vi "Celda solar Tiempo Real.vi"() -> ()   [LabVIEW 2014]
uses:
  <vilib>/imath/engines/lvmath2/RunTimeEngine/ArithmeticOperatorToken/NIMS_ArithmeticOperator_power(S).vi
  <instcachedir>/0/NIMS_ArithmeticOperator_power(S)_CAFE680B12A64A3A8F5E28A20C679B7D.lvgen/NIMS_ArithmeticOperator_power(S)_CAFE680B12A64A3A8F5E28A20C679B7D_014.vi
  <vilib>/imathl/engines/lvmath/Functions/Error Handling/Create Error.vi
  <vilib>/imath/engines/lvmath2/RunTimeEngine/CommandStatement/MC_CommandStatement_break.vi
  <vilib>/imath/engines/lvmath2/RunTimeEngine/RangeToken/NIMS_Range_R2 - Integer.vi
  <instcachedir>/0/NIMS_Range_R2 - Integer_2D1304BAF97744E0A293025746CBADFC.lvgen/NIMS_Range_R2 - Integer_2D1304BAF97744E0A293025746CBADFC_000.vi
  <vilib>/imath/engines/lvmath2/RunTimeEngine/IndexReplace/NIMS V(S)=S.vi
  <instcachedir>/0/NIMS V(S)=S_2D52C4EC15D8415E870AEE69FB516CCA.lvgen/NIMS V(S)=S_2D52C4EC15D8415E870AEE69FB516CCA_001.vi
  <instcachedir>/0/NIMS V(S)=S_2D52C4EC15D8415E870AEE69FB516CCA.lvgen/NIMS V(S)=S_2D52C4EC15D8415E870AEE69FB516CCA_000.vi
  <vilib>/imath/engines/lvmath2/RunTimeEngine/CommandStatement/NIMS_CommandStatement_MaskErr.vi
  <vilib>/imath/engines/lvmath2/RunTimeEngine/NodeEndStatement/NIMS_NodeEndStatement_Output.vi
  <instcachedir>/0/NIMS_NodeEndStatement_Output_53EC0D466D134D7ABD903AC30B43404B.lvgen/NIMS_NodeEndStatement_Output_53EC0D466D134D7ABD903AC30B43404B_000.vi
  <instcachedir>/0/NIMS_NodeEndStatement_Output_53EC0D466D134D7ABD903AC30B43404B.lvgen/NIMS_NodeEndStatement_Output_53EC0D466D134D7ABD903AC30B43404B_005.vi
  <vilib>/imath/engines/lvmath2/RunTimeEngine/ErrorHandling/NIMS_Finalize Error.vi
panel:
  out "Voltaje maximo":dbl
  out "Potencia Maxima":sgl
  out "x*y":cdb[](array[numeric])
  in  "Tab Control":enum32{"Page 2"}(tab)
  in  "Retraso (ms)":i32(slide) scale=0.0..500.0
  in  "Resistencia de carga":dbl
  out "Curva de Potencia":cluster{dbl[], sgl[]}(graph)
  in  "Configuracion":enum32{"Predeterminado", "Avanzado"}(tab)
  out "Factor de calidad":dbl=1.2
  out "T1":dbl=1.2
  out "Voc T1":dbl=1.2
  out "Isc T1":dbl=1.2
  out "T2":dbl=1.2
  out "Voc T2":dbl=1.2
  out "Isc T2":dbl=1.2
  in  "Principales Marcas":u16(ring) items=["Solarex MSX60", "Jinko Solar Perc 60-JKM300M-60", "Suntech STP275S-20", "Trina Solar TSM-250PD05", "Canadian Solar CS6X-305P", "JA Solar JAM6 PR mono 60", "Hanwha Q.Peak-G4.1", "Sharp ND-F2Q235", "Yingli YGE Serie YL275P-29b", "SolarWorld SW290", "Kyocera KD265GX-LFB\""]
  out "Vg":dbl=1.2
  out "Celdas en serie":dbl
  in  "Factor de calidad":dbl
  in  "Vg":dbl
  in  "T1":dbl
  in  "Voc T1":dbl
  in  "Isc T1":dbl
  in  "T2":dbl
  in  "Voc T2":dbl
  in  "Isc T2":dbl
  in  "Celdas en series":dbl
  out "Curva Caracteristica I-V":cluster{"Vao":dbl[], "Iao":dbl[]}[](graph)
  out "?":string
  in  "stop":bool
  in  "Paneles en serie":dbl min=1.0
  in  "Paneles en paralelo":dbl min=1.0
  in  "Fecha inicial":timestamp format="%<%Y/%m/%d>T"
  in  "Fecha final":timestamp format="%<%Y/%m/%d>T"
  in  "Latitud":string="10.41"
  in  "Longitud":string="-66.88"
  in  "OK Button":bool
  out "modelo":string
  out "String":string
  out "Numeric":i32
  out "Ia":cdb[](array[numeric])
  # "Curva 1: curva característica del panel solar\n\nCurva 2: recta de carga"
  # "Curva 1: curva de potencia del panel solar"
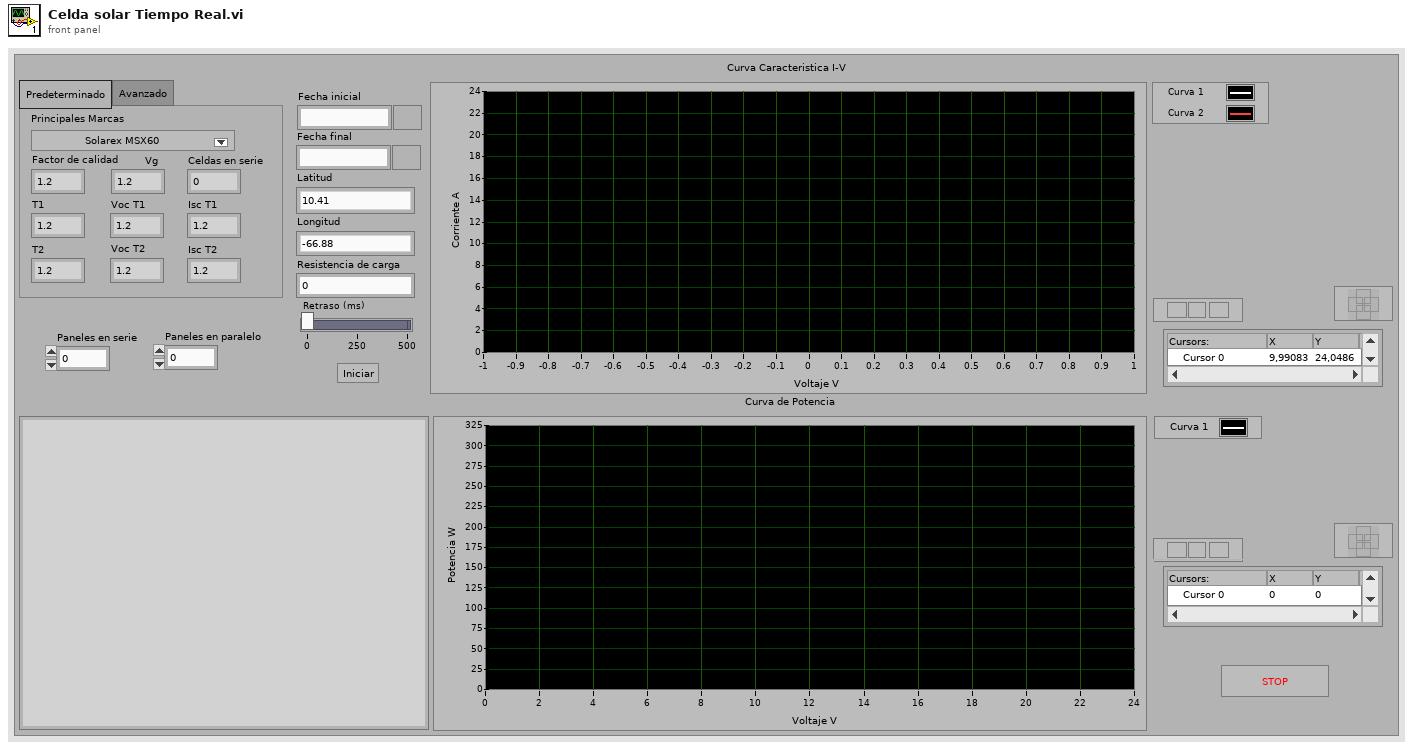
[diagram p1: front panel]
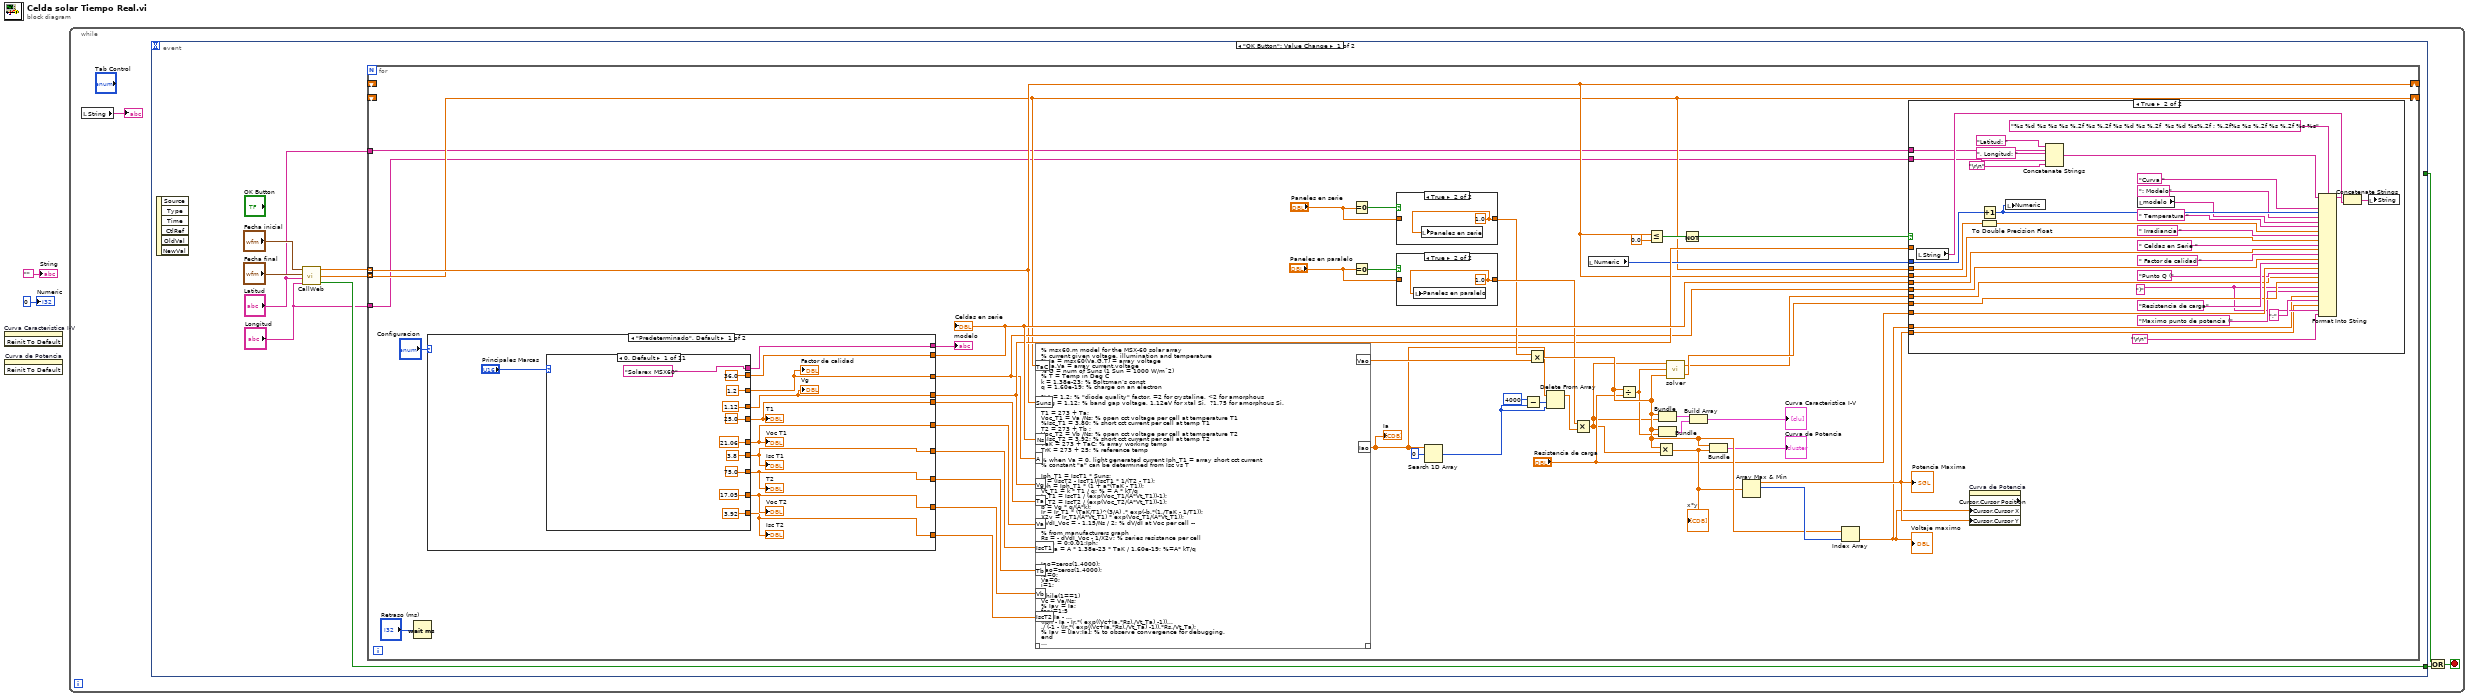
[diagram p0: block diagram]
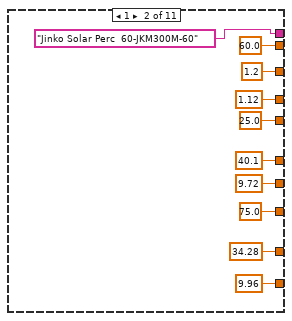
[diagram p4: hidden frame]
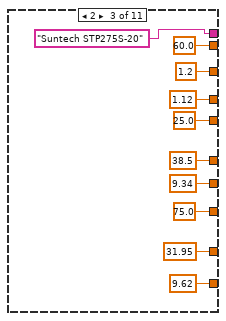
[diagram p5: hidden frame]
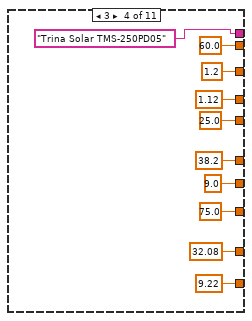
[diagram p6: hidden frame]
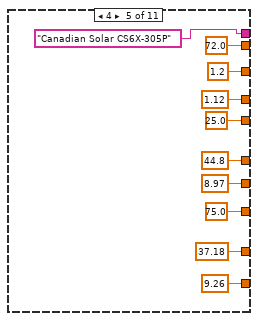
[diagram p7: hidden frame]
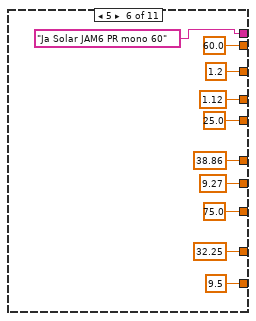
[diagram p8: hidden frame]
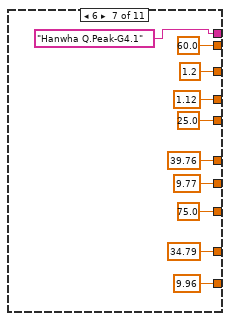
[diagram p9: hidden frame]
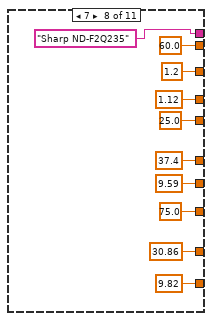
[diagram p10: hidden frame]
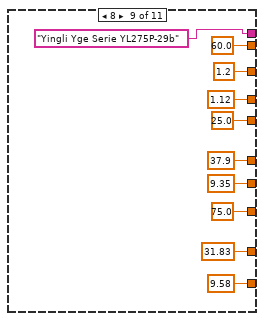
[diagram p11: hidden frame]
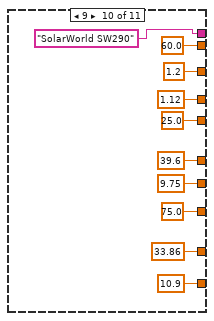
[diagram p12: hidden frame]
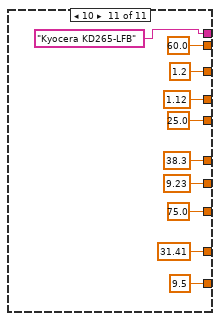
[diagram p13: hidden frame]
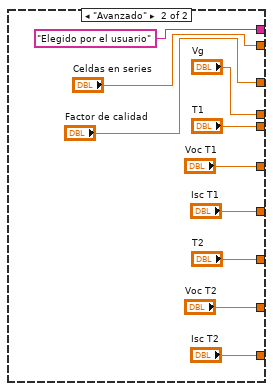
[diagram p14: hidden frame]
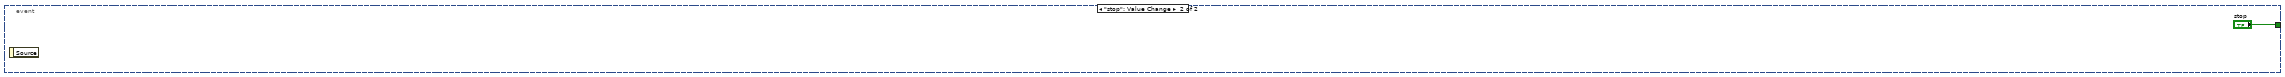
[diagram p16: hidden frame]
diagram:
  n1 = invoke on="Curva Caracteristica I-V" class="XYGraph (strict)" method="Reinit To Default"() -> ()  [unwired: 3 in, 3 out]
  n2 = invoke on="Curva de Potencia" class="XYGraph (strict)" method="Reinit To Default"() -> ()  [unwired: 3 in, 3 out]
  n3 = while {
    stop <- w4 stop-if-true
    n4 = local read "String"() -> (→"?":string)
    n5 = event shown="[0] \"OK Button\": Value Change" {
      selector: _ -> [_ _]
      dyn-events: _ -> [_ _]
      timeout: _ -> [_ _]
      tunnel: [_ "stop"] -> w6
      tunnel: [w9 _] -> w5
      event "OK Button": Value Change {
        n6 = event-data() -> ()  [unwired: 1 in, 6 out]
        n7 = call "CallWeb.vi"("Longitud"="Longitud", "Latitud"="Latitud", "Fecha final"="Fecha final", "Fecha inicial"="Fecha inicial") -> ("error?"=w9:bool, "temperatura"=w10:dbl[], "irradiancia"=w11:dbl[])  [unwired: 1 out]
        n8 = for {
          tunnel: w11 -> [w18] mode=indexing
          shift-right: [w17] -> _
          shift-left: _ -> [_]
          shift-right: [w18] -> _
          shift-left: _ -> [_]
          tunnel: w10 -> [w17] mode=indexing
          tunnel: "Latitud" -> [w15]
          tunnel: "Longitud" -> [w14]
          n9 = Wait (ms)(milliseconds to wait="Retraso (ms)") -> ()  [unwired: 1 out]
          n10 = case shown="\"Predeterminado\", Default" "Configuracion" {
            tunnel: [w74 "Factor de calidad"] -> w26
            tunnel: [w73 "Vg"] -> w27
            tunnel: [w72 "T1"] -> w32
            tunnel: [w71 "Voc T1"] -> w28
            tunnel: [w70 "Isc T1"] -> w33
            tunnel: [w69 "T2"] -> w29
            tunnel: [w68 "Voc T2"] -> w30
            tunnel: [w67 "Isc T2"] -> w31
            tunnel: [w66 "Celdas en series"] -> w60
            tunnel: [w65 "Elegido por el usuario"] -> w35
            frame "Predeterminado", Default {
              n11 = case shown="0, Default" "Principales Marcas" {
                tunnel: [1.2 1.2 1.2 1.2 1.2 1.2 1.2 1.2 1.2 1.2 1.2] -> w74
                tunnel: [1.12 1.12 1.12 1.12 1.12 1.12 1.12 1.12 1.12 1.12 1.12] -> w73
                tunnel: [25.0 25.0 25.0 25.0 25.0 25.0 25.0 25.0 25.0 25.0 25.0] -> w72
                tunnel: [21.06 40.1 38.5 38.2 44.8 38.86 39.76 37.4 37.9 39.6 38.3] -> w71
                tunnel: [3.8 9.72 9.34 9.0 8.97 9.27 9.77 9.59 9.35 9.75 9.23] -> w70
                tunnel: [75.0 75.0 75.0 75.0 75.0 75.0 75.0 75.0 75.0 75.0 75.0] -> w69
                tunnel: [17.05 34.28 31.95 32.08 37.18 32.25 34.79 30.86 31.83 33.86 31.41] -> w68
                tunnel: [3.92 9.96 9.62 9.22 9.26 9.5 9.96 9.82 9.58 10.9 9.5] -> w67
                tunnel: [36.0 60.0 60.0 60.0 72.0 60.0 60.0 60.0 60.0 60.0 60.0] -> w66
                tunnel: ["Solarex MSX60" "Jinko Solar Perc  60-JKM300M-60" "Suntech STP275S-20" "Trina Solar TMS-250PD05" "Canadian Solar CS6X-305P" "Ja Solar JAM6 PR mono 60" "Hanwha Q.Peak-G4.1" "Sharp ND-F2Q235" "Yingli Yge Serie YL275P-29b" "SolarWorld SW290" "Kyocera KD265-LFB"] -> w65
                frame 0, Default {
                }
                frame 1 {
                }
                frame 2 {
                }
                frame 3 {
                }
                frame 4 {
                }
                frame 5 {
                }
                frame 6 {
                }
                frame 7 {
                }
                frame 8 {
                }
                frame 9 {
                }
                frame 10 {
                }
              }
              "Factor de calidad" <- w74
              "Vg" <- w73
              "T1" <- w72
              "Voc T1" <- w71
              "Isc T1" <- w70
              "T2" <- w69
              "Voc T2" <- w68
              "Isc T2" <- w67
            }
            frame "Avanzado" {
            }
          }
          "Celdas en serie" <- w60
          "modelo" <- w35
          n12 = mathscript code="% msx60.m model for the MSX-60 solar array\n% current given voltage, illumination and temperature\n% Ia = msx60(Va,G,T) = array voltage\n% Ia,Va = array current,voltage\n% G = num of Suns (1 Sun = 1000 W/mˆ2)\n% T = Temp in Deg C\nk = 1.38e-23; % Boltzman’s const\nq = 1.60e-19; % charge on an electron\n\n%A = 1.2; % \"diode quality\" factor, =2 for crystaline, <2 for amorphous\n%Vg = 1.12; % band gap voltage, 1.12eV for xtal Si,  ?1.75 for amorphous Si.\n\nT1 = 273 + Ta;\nVoc_T1 = Va /Ns; % open cct voltage per cell at temperature T1\n%Isc_T1 = 3.80; % short cct current per cell at temp T1\nT2 = 273 + Tb ;\nVoc_T2 = Vb /Ns; % open cct voltage per cell at temperature T2\n%Isc_T2 = 3.92; % short cct current per cell at temp T2\nTaK = 273 + TaC; % array working temp\nTrK = 273 + 25; % reference temp\n\n% when Va = 0, light generated current Iph_T1 = array short cct current\n% constant \"a\" can be determined from Isc vs T\n\nIph_T1 = IscT1 * Suns;\na = (IscT2 - IscT1)/IscT1 * 1/(T2 - T1);\nIph = Iph_T1 * (1 + a*(TaK - T1));\nVt_T1 = k * T1 / q; % = A * kT/q\nIr_T1 = IscT1 / (exp(Voc_T1/(A*Vt_T1))-1);\nIr_T2 = IscT2 / (exp(Voc_T2/(A*Vt_T1))-1);\nb = Vg * q/(A*k);\nIr = Ir_T1 * (TaK/T1)^(3/A) .* exp(-b.*(1./TaK - 1/T1));\nX2v = Ir_T1/(A*Vt_T1) * exp(Voc_T1/(A*Vt_T1));\ndVdI_Voc = - 1.15/Ns / 2; % dV/dI at Voc per cell --\n\n% from manufacturers graph\nRs = - dVdI_Voc - 1/X2v; % series resistance per cell\n% Ia = 0:0.01:Iph;\nVt_Ta = A * 1.38e-23 * TaK / 1.60e-19; %=A* kT/q\n\n\nIao=zeros(1,4000);\nVao=zeros(1,4000);\nIa=0;\nVa=0;\ni=1;\n\nwhile(1==1)\nVc = Va/Ns;\n% Iav = Ia;\nfor j=1:5\nIa= Ia - ...\n(Iph - Ia - Ir.*( exp((Vc+Ia.*Rs)./Vt_Ta) -1))...\n./ (-1 - (Ir.*( exp((Vc+Ia.*Rs)./Vt_Ta) -1)).*Rs./Vt_Ta);\n% Iav = [Iav;Ia]; % to observe convergence for debugging.\nend\n\nif(Ia<=0) break\nend\n\nIao(i)=Ia;\nVao(i)=Va;\n\ni=i+1;\nVa=Va+1/100;\n\nend"("TaC"=w17, "Suns"=w18, "Ns"=w60, "Vg"=w27, "A"=w26, "Ta"=w32, "Va"=w28, "IscT1"=w33, "Tb"=w29, "Vb"=w30, "IscT2"=w31) -> ("Iao"=w36:cdb[], "Vao"=w38:dbl[])  [unwired: 1 in, 1 out]
          "Ia" <- w36
          n13 = Equal To 0?(x="Paneles en serie") -> (x = 0?=w39:bool)
          n14 = Equal To 0?(x="Paneles en paralelo") -> (x = 0?=w41:bool)
          n15 = case shown="True" w39 {
            tunnel: [w63 w64] -> w40
            tunnel: "Paneles en serie" -> [w63 _]
            frame False {
            }
            frame True {
              w64 = 1.0
              n16 = local write "Paneles en serie"(w64) -> ()
            }
          }
          n17 = case shown="True" w41 {
            tunnel: [w61 w62] -> w42
            tunnel: "Paneles en paralelo" -> [w61 _]
            frame False {
            }
            frame True {
              w62 = 1.0
              n18 = local write "Paneles en paralelo"(w62) -> ()
            }
          }
          n19 = Search 1D Array(1D array=w36, element=0) -> (index of element=w22:i32)  [unwired: 1 in]
          n20 = Subtract(x=4000, y=w22) -> (x-y=w21:i32)
          n21 = Multiply(x=w40, y=w38) -> (x*y=w54:dbl[])
          n22 = Delete From Array(array=w36, length=w21, index=w22) -> (array with subset deleted=w37:cdb[])  [unwired: 1 out]
          n23 = Multiply(x=w42, y=w37) -> (x*y=w43:cdb[])
          n24 = local read "Numeric"() -> (w25:i32)
          n25 = Divide(x=w54, y="Resistencia de carga") -> (x/y=w44:dbl[])
          n26 = Less Or Equal?(x=w18, y=0.0) -> (x <= y?=w51:bool)
          n27 = Multiply(x=w54, y=w43) -> (x*y=w53:sgl[])
          "x*y" <- w53
          n28 = Bundle(w54, w43) -> (w23:cluster{dbl[], cdb[]})  [unwired: 1 in]
          n29 = Bundle(w54, w44) -> (w45:cluster{dbl[], dbl[]})  [unwired: 1 in]
          n30 = call "solver.vi"("Voltaje"=w54, "Ec 2"=w44, "Ec 1"=w43) -> ("y"=w47:dbl, "x"=w46:dbl)
          n31 = Not(x=w51) -> (.not. x?=w52:bool)
          n32 = Build Array(w23, w45) -> (→"Curva Caracteristica I-V":cluster{dbl[], cdb[]}[])
          n33 = Bundle(w54, w53) -> (→"Curva de Potencia":cluster{dbl[], sgl[]})  [unwired: 1 in]
          n34 = Array Max & Min(array=w53) -> (max value=w57:sgl, max index (indices)=w55:i32)  [unwired: 2 out]
          "Potencia Maxima" <- w57
          n35 = Index Array(array=w54, index=w55) -> (element=w56:dbl)
          "Voltaje maximo" <- w56
          n36 = case shown="True" w52 {
            tunnel: w25 -> [_ w749]
            tunnel: w17 -> [_ w734]
            tunnel: w18 -> [_ w743]
            tunnel: w60 -> [_ w741]
            tunnel: w26 -> [_ w739]
            tunnel: w27 -> [_ _]
            tunnel: w46 -> [_ w730]
            tunnel: w47 -> [_ w729]
            tunnel: "Resistencia de carga" -> [_ w732]
            tunnel: w57 -> [_ w724]
            tunnel: w56 -> [_ w725]
            tunnel: w15 -> [_ w717]
            tunnel: w14 -> [_ w716]
            frame False {
            }
            frame True {
              w726 = ")"
              n37 = local read "String"() -> (w723:string)
              n38 = Increment(x=w749) -> (x+1=w747:i32)
              n39 = To Double Precision Float(number=w734) -> (double precision float=w735:dbl)
              n40 = local write "Numeric"(w747) -> ()
              n41 = Concatenate Strings("Latitud: ", w717, ", Longitud: ", w716, "\r\n") -> (w715:string)
              n42 = local read "modelo"() -> (w736:string)
              n43 = Format Into String(format string="%s %d %s %s %s %.2f %s %.2f %s %d %s %.2f  %s %d %s%.2f ; %.2f%s %s %.2f %s %.2f %s %s", initial string=w715, "Curva ", w747, ": Modelo", w736, " Temperatura ", w735, " Irradiancia ", w743, " Celdas en Serie ", w741, " Factor de calidad ", w739, "Resistencia de carga", w732, "Punto Q (", w730, w729, w726, "Maximo punto de potencia (", w725, ";", w724, w726, "\r\n") -> (resulting string=w748:string)  [unwired: 1 in, 1 out]
              n44 = Concatenate Strings(w723, w748) -> (w746:string)
              n45 = local write "String"(w746) -> ()
            }
          }
          n46 = property on="Curva de Potencia" class="XYGraph (strict)" props=["Cursor", "Cursor Position", "Cursor", "Cursor X", "Cursor", "Cursor Y"]("Cursor.Cursor X"=w56, "Cursor.Cursor Y"=w57) -> ()  [unwired: 2 in, 3 out]
        }
      }
      event "stop": Value Change {
        n47 = event-data() -> ()  [unwired: 1 in, 1 out]
      }
    }
    n48 = Or(x=w6, y=w5) -> (x .or. y?=w4:bool)
  }
  "Numeric" <- 0
  "String" <- ""
